vi "from_file_open.vi"(5 "Reset":bool, 6 "Add Bit Padding":bool, 7 "error in (no error)":errorcluster, 8 "Guard Bits to Add":i32=32, 9 "M-ary (16)":i32=16 step=2, 10 "InputStrig":string) -> (0 "error out":errorcluster, 1 "Guard Bits Added":i32, 2 "Character Array":u8[](array[numeric]), 3 "Bitstream (with Guard Bits)":i8[](array[numeric]), 4 "Pure Bit Stream":i8[](array[numeric]))   [LabVIEW 2019]
uses:
  <vilib>/addons/Modulation/Digital/Support/Common/Validators/mod_Generate Bits Validate.vi
  <vilib>/addons/Modulation/Digital/General/subVIs/mod_Generate Bits Pattern.vi
  <vilib>/addons/Modulation/Analog/support/mod_Set Error Source.vi
  <vilib>/addons/Modulation/Digital/General/subVIs/mod_Generate Bits PN Sequence.vi
  <vilib>/addons/Modulation/niDMT.lvlib
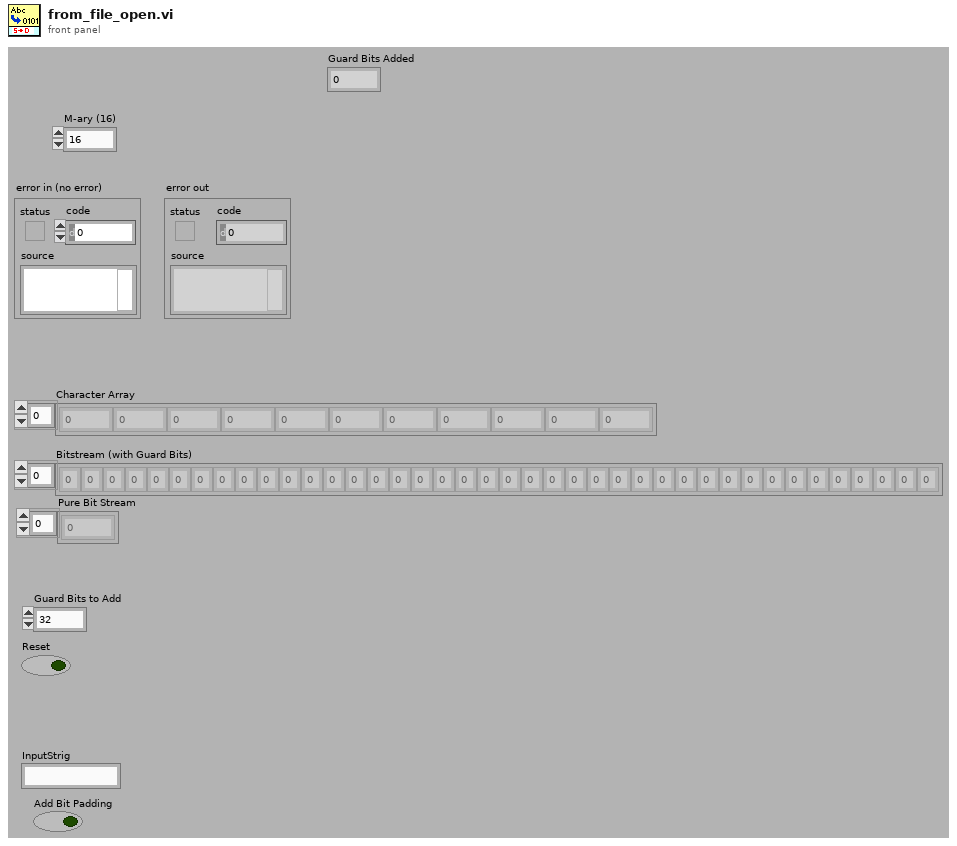
[diagram p1: front panel]
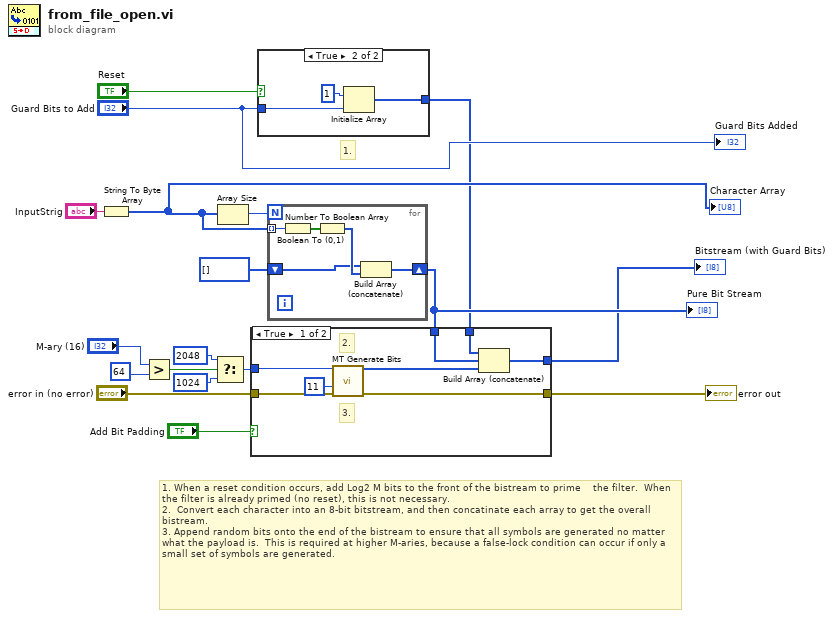
[diagram p0: block diagram]
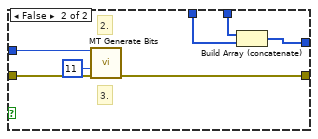
[diagram p2: hidden frame]
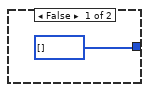
[diagram p3: hidden frame]
diagram:
  # "1."
  # "1. When a reset condition occurs, add Log2 M bits to the front of the bistream to prime    the filter.  When the filter is already primed (no reset), this is not necessary.\n2.  Convert each character into an 8-bit bitstream, and then concatinate each array to get the overall bistream.\n3. Append random bits onto the end of the bistream to ensure that all symbols are generated no matter what the payload is.  This is required at higher M-aries, because a false-lock condition can occur if only a small set of symbols are generated."
  n1 = String To Byte Array(string="InputStrig") -> (unsigned byte array=w14:u8[])
  "Character Array" <- w14
  n2 = Greater?(x="M-ary (16)", y=64) -> (0:w7:bool)
  n3 = Select(t=2048 ("total bits (128)"), s=w7, f=1024 ("total bits (128)")) -> (s? t:f=w3:i32)
  n4 = Array Size(array=w14) -> (size(s)=w9:i32)
  n5 = case shown="True" "Reset" {
    tunnel: [i32[] [] w21] -> w8
    tunnel: "Guard Bits to Add" -> [_ w20]
    frame False {
    }
    frame True {
      n6 = Initialize Array(1 ("new element/subarray"), w20) -> (w21:i32[])
    }
  }
  n7 = for {
    N: w9 -> [_]
    shift-right: [w23] -> w18
    shift-left: i8[] [] -> [w24]
    tunnel: w14 -> [w26] mode=indexing
    n8 = Number To Boolean Array(number=w26) -> (Boolean array=w27:bool[])
    n9 = Boolean To (0,1)(Boolean=w27) -> (0, 1=w25:i16[])
    n10 = Build Array (concatenate)(w24, w25) -> (w23:i16[])
  }
  "Pure Bit Stream" <- w18
  n11 = case shown="True" "Add Bit Padding" {
    tunnel: w18 -> [w35 w42]
    tunnel: [w34 w41] -> w13
    tunnel: "error in (no error)" -> [w33 w40]
    tunnel: [w32 w39] -> w11
    tunnel: w8 -> [w31 w38]
    tunnel: w3 -> [w28 w36]
    frame True {
      # "2."
      # "3."
      n12 = call <vilib>:"MT Generate Bits.vi"("total bits (128)"=w28, "PN sequence order (9)"=11, "error in (no error)"=w33) -> ("output bit stream"=w29:i8[], "error out"=w32:errorcluster)  [unwired: 5 in, 6 out]
      n13 = Build Array (concatenate)(w31, w35, w29) -> (w34:i32[])
    }
    frame False {
      # "2."
      # "3."
      n14 = call <vilib>:"MT Generate Bits.vi"("total bits (128)"=w36, "PN sequence order (9)"=11, "error in (no error)"=w40) -> ("error out"=w39:errorcluster)  [unwired: 5 in, 7 out]
      n15 = Build Array (concatenate)(w38, w42) -> (w41:i32[])
    }
  }
  "error out" <- w11
  "Bitstream (with Guard Bits)" <- w13
  "Guard Bits Added" <- "Guard Bits to Add"
